vi "Process Menu.vi"(0 "Listbox":refnum<vi>, 1 "Default":string[](array[string]), 5 "menu tag":string, 7 "Row":i32, 9 "Properties":T3, 11 "error in (no error)":errorcluster, 12 "Columns":T1[](array[typedef])) -> (6 "Event type":T4, 8 "Row Out":i32, 10 "data changed?":bool, 15 "error out":errorcluster)   [LabVIEW 2020, in "KTable.xctl"]
uses:
  KTable.xctl
  Event Type.ctl
  Table Properties.ctl
  ColumnSpec.ctl
  ColumnType.ctl
  Array Manipulation VIs/Array-Dimensions (2D string).vi
panel:
  out "Listbox Out":refnum<vi>
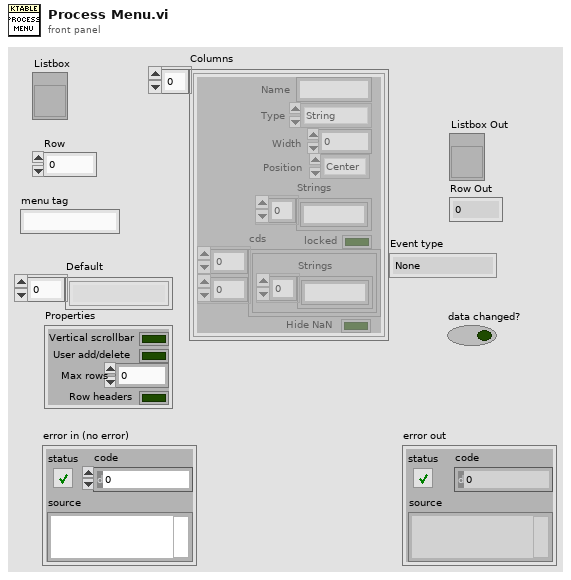
[diagram p1: front panel]
types:
  T1 = typedef "KTable.xctl/ColumnSpec.ctl" = cluster{"Name":string, "Type":T2, "Width":i32, "Strings":string[], "Position":enum16{"Left", "Center", "Right"}, "locked":bool, "cds":cluster{"Strings":string[]}[][], "Hide NaN":bool}
  T2 = typedef "KTable.xctl/ColumnType.ctl" = enum16{"String", "Enum", "Int", "Double", "Boolean", "Ring", "Formula", "Color"}
  T3 = typedef "KTable.xctl/Table Properties.ctl" = cluster{"Vertical scrollbar":bool, "User add/delete":bool, "Max rows":i32, "Row headers":bool}
  T4 = typedef "KTable.xctl/Event Type.ctl" = enum16{"None", "Selection", "Edit", "Insert", "Delete", "Up", "Down", "Duplicate"}
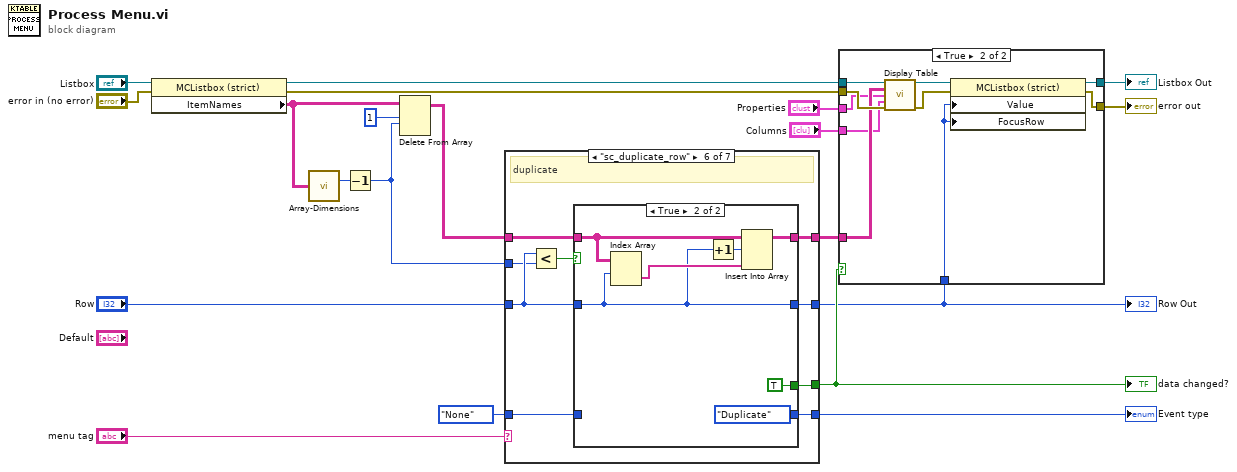
[diagram p0: block diagram]
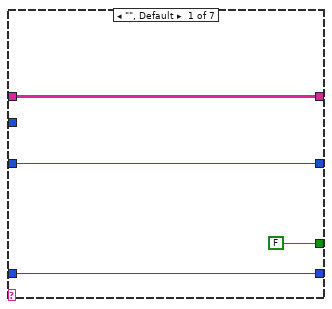
[diagram p2: hidden frame]
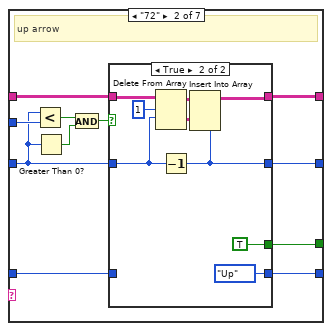
[diagram p3: hidden frame]
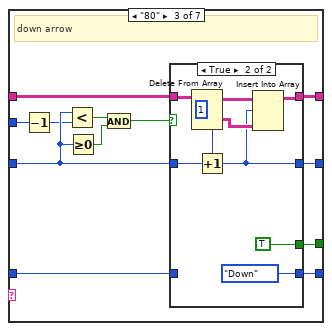
[diagram p5: hidden frame]
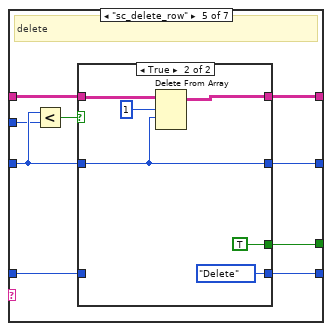
[diagram p8: hidden frame]
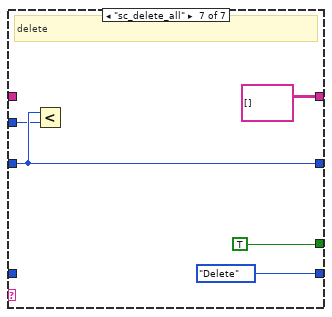
[diagram p11: hidden frame]
diagram:
  n1 = property class="MCListbox (strict)"(reference="Listbox", error in="error in (no error)") -> (reference out=w16:refnum<vi>, error out=w14:errorcluster, "ItemNames"=w8:string[][])
  n2 = call-poly "Array-Dimensions.vi"("2D Array"=w8) -> ("# rows"=w7:i32)  [unwired: 13 in, 1 out]
  n3 = Decrement(x=w7) -> (x-1=w6:i32)
  n4 = Delete From Array(array=w8, length=1, index (row)=w6) -> (array with subset deleted=w10:string[][])  [unwired: 1 in, 1 out]
  n5 = case shown="\"sc_duplicate_row\"" "menu tag" {
    tunnel: [FALSE w31 w55 _ w78 w96 TRUE] -> w15
    tunnel: "Row" -> [w23 w28 w52 w73 w81 w99 w116]
    tunnel: w10 -> [w22 w35 w59 w74 w83 w101 _]
    tunnel: w6 -> [_ w30 w54 _ w77 w95 w114]
    tunnel: [w23 w33 w57 w73 w80 w98 w116] -> w5
    tunnel: [w22 w32 w56 w74 w79 w97 string[][] [] ("ItemNames")] -> w11
    tunnel: Event_Type."None" ("Type") -> [w21 w26 w49 w72 w75 w93 _]
    tunnel: [w21 w25 w48 w72 w76 w94 Event_Type."Delete" ("Type")] -> w3
    frame "", Default {
    }
    frame "72" {
      # "up arrow"
      n6 = Less?(x=w28, y=w30) -> (x < y?=w34:bool)
      n7 = Greater Than 0?(x=w28) -> (x > 0?=w27:bool)
      n8 = And(x=w34, y=w27) -> (x .and. y?=w29:bool)
      n9 = case shown="True" w29 {
        tunnel: w35 -> [w37 w47]
        tunnel: w28 -> [w38 w45]
        tunnel: [w37 w41] -> w32
        tunnel: [w38 w40] -> w33
        tunnel: [_ TRUE] -> w31
        tunnel: w26 -> [w36 _]
        tunnel: [w36 Event_Type."Up" ("Type")] -> w25
        frame False {
        }
        frame True {
          n10 = Delete From Array(array=w47, length=1, index (row)=w45) -> (deleted portion=w42:string[][], array with subset deleted=w43:string[][])  [unwired: 1 in]
          n11 = Decrement(x=w45) -> (x-1=w40:i32)
          n12 = Insert Into Array(array=w43, index (row)=w40, new element=w42) -> (w41:string[][])  [unwired: 1 in]
        }
      }
    }
    frame "80" {
      # "down arrow"
      n13 = Decrement(x=w54) -> (x-1=w50:i32)
      n14 = Less?(x=w52, y=w50) -> (x < y?=w58:bool)
      n15 = Greater Or Equal To 0?(x=w52) -> (x >= 0?=w51:bool)
      n16 = And(x=w58, y=w51) -> (x .and. y?=w53:bool)
      n17 = case shown="True" w53 {
        tunnel: w59 -> [w61 w71]
        tunnel: w52 -> [w62 w69]
        tunnel: [w61 w65] -> w56
        tunnel: [w62 w64] -> w57
        tunnel: [_ TRUE] -> w55
        tunnel: w49 -> [w60 _]
        tunnel: [w60 Event_Type."Down" ("Type")] -> w48
        frame False {
        }
        frame True {
          n18 = Delete From Array(array=w71, length=1, index (row)=w69) -> (deleted portion=w66:string[][], array with subset deleted=w67:string[][])  [unwired: 1 in]
          n19 = Increment(x=w69) -> (x+1=w64:i32)
          n20 = Insert Into Array(array=w67, index (row)=w64, new element=w66) -> (w65:string[][])  [unwired: 1 in]
        }
      }
    }
    frame "82" {
      # "insert"
    }
    frame "sc_delete_row" {
      # "delete"
      n21 = Less?(x=w81, y=w77) -> (x < y?=w82:bool)
      n22 = case shown="True" w82 {
        tunnel: w83 -> [w85 w92]
        tunnel: w81 -> [w86 w89]
        tunnel: [w85 w90] -> w79
        tunnel: [w86 w89] -> w80
        tunnel: [_ TRUE] -> w78
        tunnel: [w84 Event_Type."Delete" ("Type")] -> w76
        tunnel: w75 -> [w84 _]
        frame False {
        }
        frame True {
          n23 = Delete From Array(array=w92, length=1, index (row)=w89) -> (array with subset deleted=w90:string[][])  [unwired: 1 in, 1 out]
        }
      }
    }
    frame "sc_duplicate_row" {
      # "duplicate"
      n24 = Less?(x=w99, y=w95) -> (x < y?=w100:bool)
      n25 = case shown="True" w100 {
        tunnel: w101 -> [w103 w109]
        tunnel: w99 -> [w104 w105]
        tunnel: [w103 w108] -> w97
        tunnel: [w104 w105] -> w98
        tunnel: [_ TRUE] -> w96
        tunnel: [w102 Event_Type."Duplicate" ("Type")] -> w94
        tunnel: w93 -> [w102 _]
        frame False {
        }
        frame True {
          n26 = Index Array(array=w109, index (row)=w105) -> (element=w106:string[])  [unwired: 1 in]
          n27 = Increment(x=w105) -> (x+1=w107:i32)
          n28 = Insert Into Array(array=w109, index (row)=w107, new element=w106) -> (w108:string[][])  [unwired: 1 in]
        }
      }
    }
    frame "sc_delete_all" {
      # "delete"
      n29 = Less?(x=w116, y=w114) -> ()  [unwired: 1 out]
    }
  }
  "data changed?" <- w15
  "Row Out" <- w5
  "Event type" <- w3
  n30 = case shown="True" w15 {
    tunnel: w16 -> [w118 w128]
    tunnel: w14 -> [w117 w127]
    tunnel: [w118 w123] -> w13
    tunnel: [w117 w122] -> w12
    tunnel: w11 -> [_ w126]
    tunnel: w5 -> [_ w121]
    tunnel: "Properties" -> [_ w120]
    tunnel: "Columns" -> [_ w119]
    frame False {
    }
    frame True {
      n31 = call "Display Table.vi"("Listbox"=w128, "Table Items"=w126, "Properties"=w120, "Columns"=w119, "error in (no error)"=w127) -> ("reference out"=w125:refnum<vi>, "error out"=w124:errorcluster)  [unwired: 9 in]
      n32 = property class="MCListbox (strict)"(reference=w125, error in=w124, "Value"=w121, "FocusRow"=w121) -> (reference out=w123:refnum<vi>, error out=w122:errorcluster)
    }
  }
  "error out" <- w12
  "Listbox Out" <- w13
